vi "smff-setpoint-state-machine.vi"(8 "Time pass through":dbl=-1.0) -> (0 "State":i32, 3 "Speed Setpoint Ft/Sec":dbl)   [LabVIEW 2019]
uses:
  <vilib>/Utility/semaphor.llb/Obtain Semaphore Reference.vi
  <vilib>/Rock Robotics/WPI/ThirdParty/JAS_Junk/TrajLib/Timer_Reset.vi
  <vilib>/Rock Robotics/WPI/ThirdParty/JAS_Junk/TrajLib/Trajectory_Library.lvlib
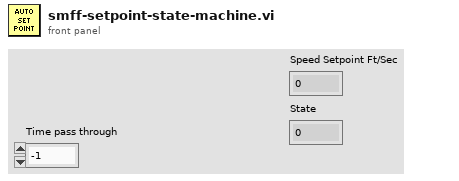
[diagram p1: front panel]
types:
  T1 = typedef "Trajectory_Library.lvlib/TIMER.ctl" = cluster{"StartTime":dbl, "Accumulated TIme":dbl, "Running":bool, "semaphore":T2}
  T2 = typedef "Semaphore RefNum" = refnum<k1>
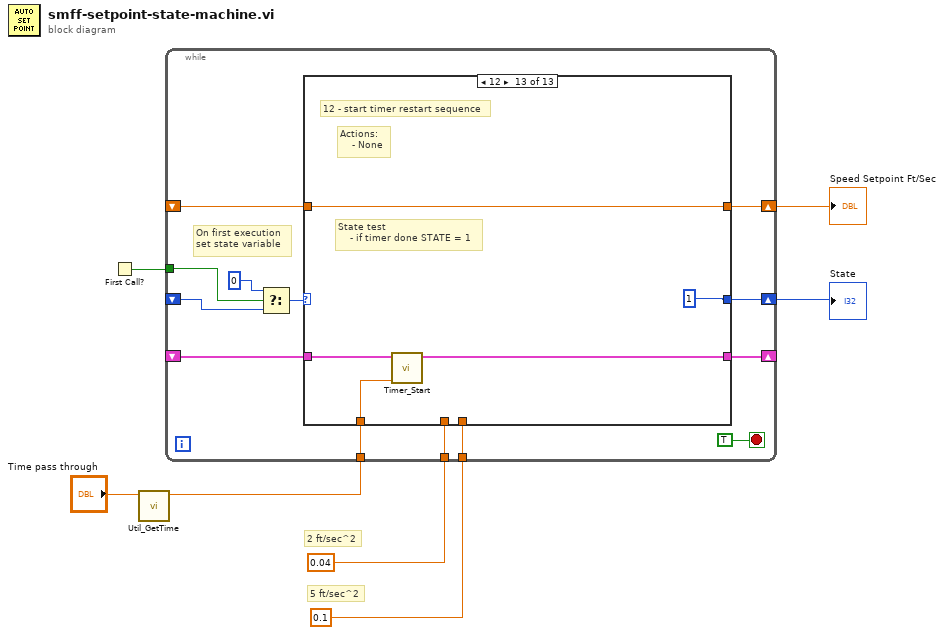
[diagram p0: block diagram]
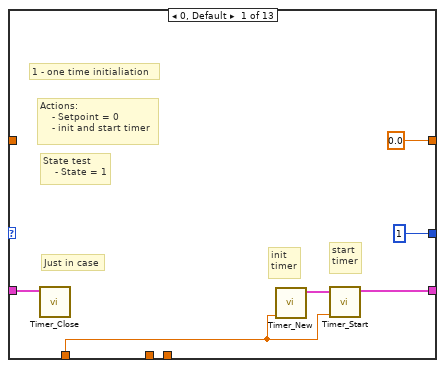
[diagram p2: hidden frame]
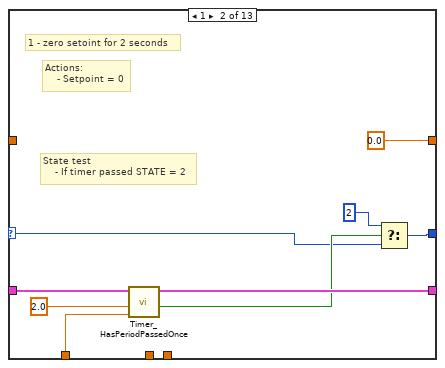
[diagram p3: hidden frame]
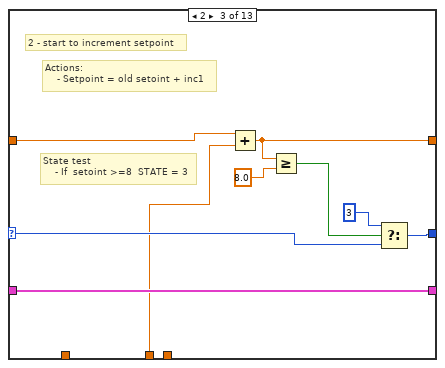
[diagram p4: hidden frame]
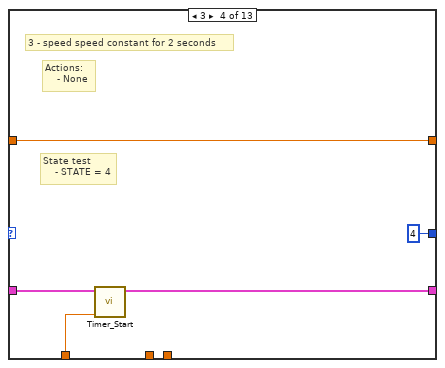
[diagram p5: hidden frame]
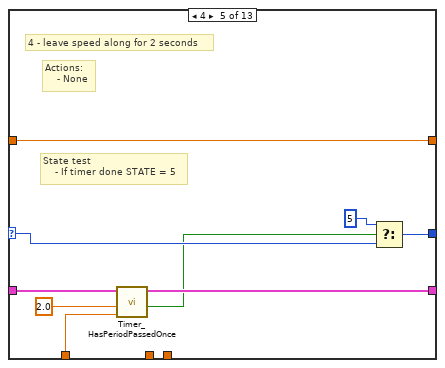
[diagram p6: hidden frame]
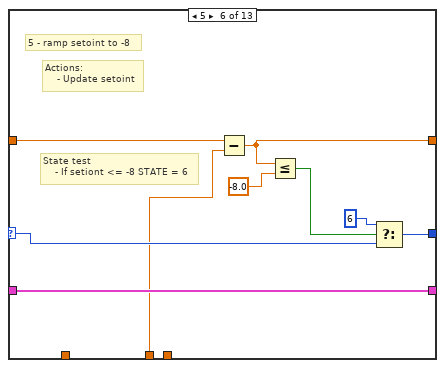
[diagram p7: hidden frame]
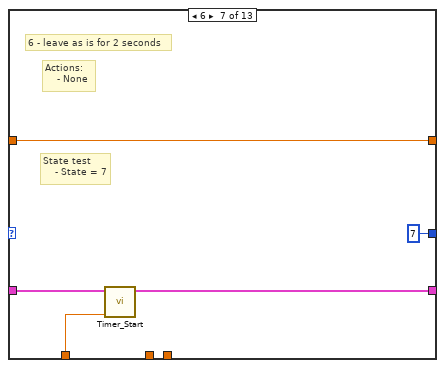
[diagram p8: hidden frame]
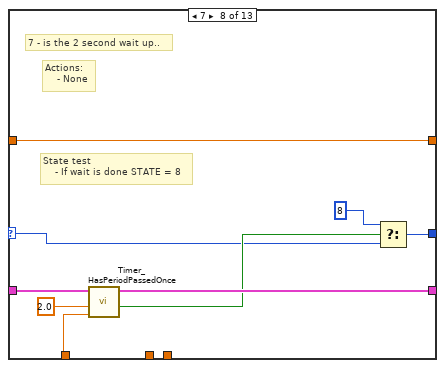
[diagram p9: hidden frame]
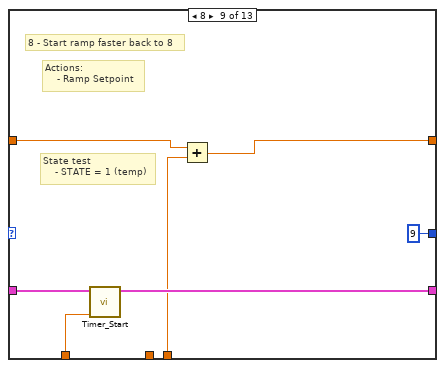
[diagram p10: hidden frame]
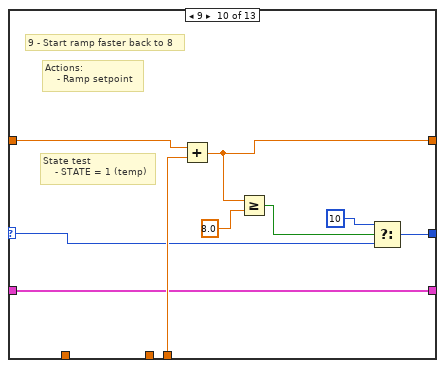
[diagram p11: hidden frame]
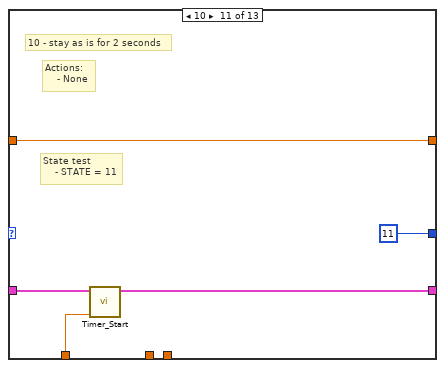
[diagram p12: hidden frame]
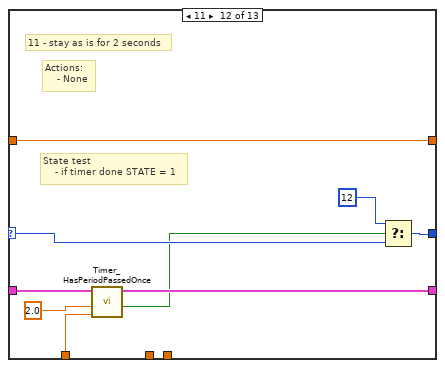
[diagram p13: hidden frame]
diagram:
  # "5 ft/sec^2"
  # "2 ft/sec^2"
  n1 = First Call?() -> (First Call?: T/F=w5:bool)
  n2 = call <vilib>:"Util_GetTime.vi"("Pass_Through_Time"="Time pass through") -> ("FPGA_Time_Seconds"=w4:dbl)  [unwired: 9 in, 1 out]
  n3 = while {
    shift-right: [w19] -> w6
    shift-left: _ -> [w17]
    tunnel: w5 -> [w16]
    shift-right: [w14] -> _
    shift-left: _ -> [w13]
    tunnel: w4 -> [w12]
    shift-right: [w11] -> w3
    shift-left: _ -> [w10]
    tunnel: 0.04 -> [w9]
    tunnel: 0.1 -> [w8]
    stop <- TRUE stop-if-true
    # "On first execution\nset state variable"
    n4 = Select(t=0, s=w16, f=w17) -> (s? t:f=w18:i32)
    n5 = case shown="12" w18 {
      selector: w18 -> [_ w29 w43 _ w53 w67 _ w74 _ w92 _ w104 _]
      tunnel: [1 ("State") w31 w44 4 ("t") w52 w66 7 ("t") w76 9 ("t") w94 11 ("t") w105 1 ("t")] -> w19
      tunnel: [w24 w32 w41 w46 w57 w63 w69 w79 w87 w95 w99 w109 w114] -> w14
      tunnel: w13 -> [w23 w34 w41 w47 w56 w63 w70 w80 w88 w95 w100 w110 w115]
      tunnel: w12 -> [w22 w35 _ w45 w55 _ w68 w78 w86 _ w98 w108 w113]
      tunnel: [0.0 0.0 w38 w49 w58 w61 w71 w81 w83 w91 w102 w111 w116] -> w11
      tunnel: w10 -> [_ _ w40 w49 w58 w64 w71 w81 w84 w97 w102 w111 w116]
      tunnel: w9 -> [_ _ w39 _ _ w62 _ _ _ _ _ _ _]
      tunnel: w8 -> [_ _ _ _ _ _ _ _ w82 w96 _ _ _]
      frame 0, Default {
        # "start\ntimer"
        # "init\ntimer"
        # "Just in case"
        # "State test\n    - State = 1"
        # "Actions:\n    - Setpoint = 0\n    - init and start timer"
        # "1 - one time initialiation"
        n6 = call <vilib>:"Timer_Close.vi"("TIMER"=w23) -> ()  [unwired: 11 in]
        n7 = call <vilib>:"Timer_New.vi"("Pass_Through_Time"=w22) -> ("TIMER"=w25:T1)  [unwired: 10 in]
        n8 = call <vilib>:"Timer_Start.vi"("Pass_Through_Time"=w22, "in Timer"=w25) -> ("out Timer"=w24:T1)  [unwired: 9 in]
      }
      frame 1 {
        # "State test\n    - If timer passed STATE = 2"
        # "Actions:\n    - Setpoint = 0"
        # "1 - zero setoint for 2 seconds"
        n9 = call <vilib>:"Timer_HasPeriodPassedOnce.vi"("Pass_Through_Time"=w35, "Period"=2.0, "in Timer"=w34) -> ("Expired"=w30:bool, "out Timer"=w32:T1)  [unwired: 6 in, 1 out]
        n10 = Select(t=2, s=w30, f=w29) -> (s? t:f=w31:i32)
      }
      frame 2 {
        # "State test\n    - If  setoint >=8  STATE = 3"
        # "Actions:\n    - Setpoint = old setoint + inc1"
        # "2 - start to increment setpoint"
        n11 = Add(x=w40, y=w39) -> (x+y=w38:dbl)
        n12 = Greater Or Equal?(x=w38, y=8.0) -> (x >= y?=w36:bool)
        n13 = Select(t=3, s=w36, f=w43) -> (s? t:f=w44:i32)
      }
      frame 3 {
        # "State test\n    - STATE = 4"
        # "Actions:\n    - None"
        # "3 - speed speed constant for 2 seconds"
        n14 = call <vilib>:"Timer_Start.vi"("Pass_Through_Time"=w45, "in Timer"=w47) -> ("out Timer"=w46:T1)  [unwired: 9 in]
      }
      frame 4 {
        # "State test\n    - If timer done STATE = 5"
        # "Actions:\n    - None"
        # "4 - leave speed along for 2 seconds"
        n15 = call <vilib>:"Timer_HasPeriodPassedOnce.vi"("Pass_Through_Time"=w55, "Period"=2.0, "in Timer"=w56) -> ("Expired"=w50:bool, "out Timer"=w57:T1)  [unwired: 6 in, 1 out]
        n16 = Select(t=5, s=w50, f=w53) -> (s? t:f=w52:i32)
      }
      frame 5 {
        # "State test\n    - If setiont <= -8 STATE = 6"
        # "Actions:\n    - Update setoint"
        # "5 - ramp setoint to -8"
        n17 = Subtract(x=w64, y=w62) -> (x-y=w61:dbl)
        n18 = Less Or Equal?(x=w61, y=-8.0) -> (x <= y?=w59:bool)
        n19 = Select(t=6, s=w59, f=w67) -> (s? t:f=w66:i32)
      }
      frame 6 {
        # "State test\n    - State = 7"
        # "Actions:\n    - None"
        # "6 - leave as is for 2 seconds"
        n20 = call <vilib>:"Timer_Start.vi"("Pass_Through_Time"=w68, "in Timer"=w70) -> ("out Timer"=w69:T1)  [unwired: 9 in]
      }
      frame 7 {
        # "State test\n    - If wait is done STATE = 8"
        # "Actions:\n    - None"
        # "7 - is the 2 second wait up.."
        n21 = call <vilib>:"Timer_HasPeriodPassedOnce.vi"("Pass_Through_Time"=w78, "Period"=2.0, "in Timer"=w80) -> ("Expired"=w75:bool, "out Timer"=w79:T1)  [unwired: 6 in, 1 out]
        n22 = Select(t=8, s=w75, f=w74) -> (s? t:f=w76:i32)
      }
      frame 8 {
        # "State test\n    - STATE = 1 (temp)"
        # "Actions:\n    - Ramp Setpoint"
        # "8 - Start ramp faster back to 8"
        n23 = call <vilib>:"Timer_Start.vi"("Pass_Through_Time"=w86, "in Timer"=w88) -> ("out Timer"=w87:T1)  [unwired: 9 in]
        n24 = Add(x=w84, y=w82) -> (x+y=w83:dbl)
      }
      frame 9 {
        # "State test\n    - STATE = 1 (temp)"
        # "Actions:\n    - Ramp setpoint"
        # "9 - Start ramp faster back to 8"
        n25 = Add(x=w97, y=w96) -> (x+y=w91:dbl)
        n26 = Greater Or Equal?(x=w91, y=8.0) -> (x >= y?=w89:bool)
        n27 = Select(t=10, s=w89, f=w92) -> (s? t:f=w94:i32)
      }
      frame 10 {
        # "State test\n    - STATE = 11"
        # "Actions:\n    - None"
        # "10 - stay as is for 2 seconds"
        n28 = call <vilib>:"Timer_Start.vi"("Pass_Through_Time"=w98, "in Timer"=w100) -> ("out Timer"=w99:T1)  [unwired: 9 in]
      }
      frame 11 {
        # "State test\n    - if timer done STATE = 1"
        # "Actions:\n    - None"
        # "11 - stay as is for 2 seconds"
        n29 = call <vilib>:"Timer_HasPeriodPassedOnce.vi"("Pass_Through_Time"=w108, "Period"=2.0, "in Timer"=w110) -> ("Expired"=w103:bool, "out Timer"=w109:T1)  [unwired: 6 in, 1 out]
        n30 = Select(t=12, s=w103, f=w104) -> (s? t:f=w105:i32)
      }
      frame 12 {
        # "State test\n    - if timer done STATE = 1"
        # "Actions:\n    - None"
        # "12 - start timer restart sequence"
        n31 = call <vilib>:"Timer_Start.vi"("Pass_Through_Time"=w113, "in Timer"=w115) -> ("out Timer"=w114:T1)  [unwired: 9 in]
      }
    }
  }
  "State" <- w6
  "Speed Setpoint Ft/Sec" <- w3
